vi "Diagram - Get All Text Refs.vi"(8 "error in (no error)":errorcluster, 11 "TopLevelDiagram in":refnum<vi>) -> (0 "error out":errorcluster, 2 "TextRefs":refnum<vi>[](array[refnum]), 3 "TopLevelDiagram out":refnum<vi>)   [LabVIEW 2017, in "csmHelper-Diagram.lvlib"]
doc: "-- <b>输入控件</b> --\n\n- <b>TopLevelDiagram in</b>:\n\n\n-- <b>输出控件</b> --\n\n- <b>TextRefs</b>:\n\n- <b>TopLevelDiagram out</b>:"
uses:
  csmHelper-Diagram.lvlib
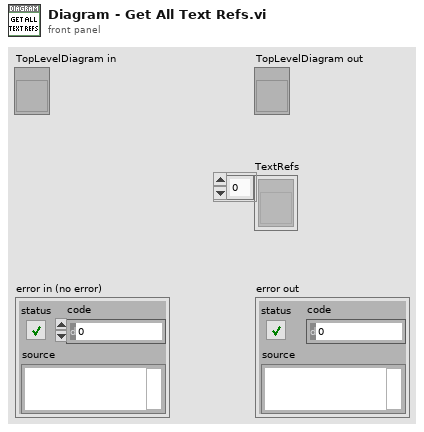
[diagram p1: front panel]
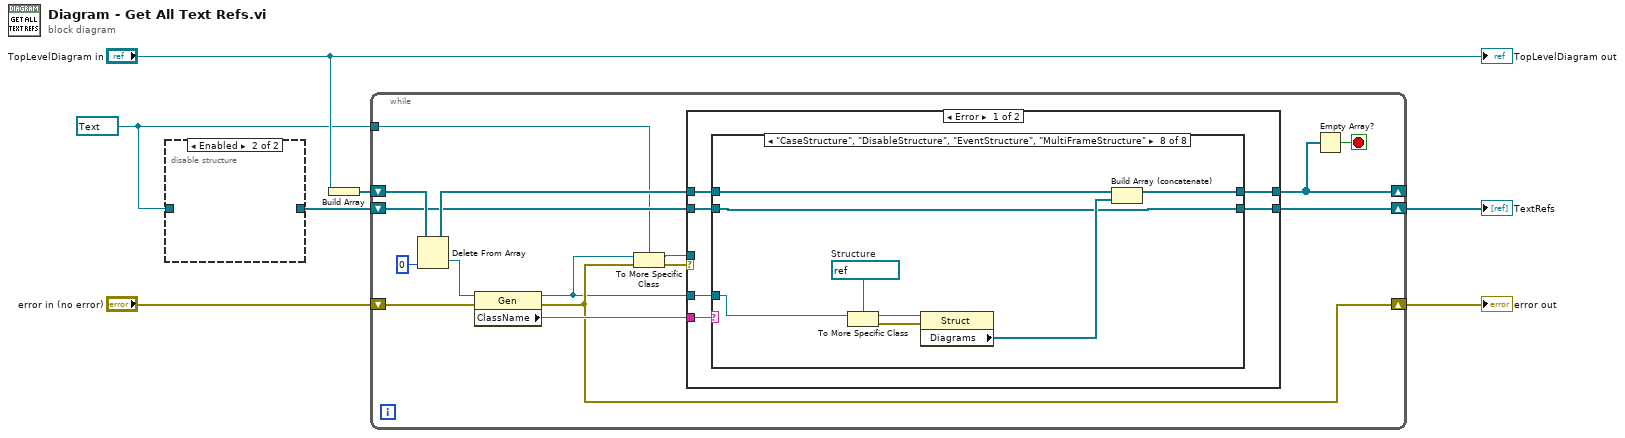
[diagram p0: block diagram]
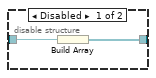
[diagram p2: hidden frame]
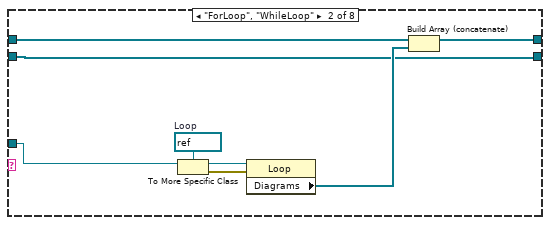
[diagram p4: hidden frame]
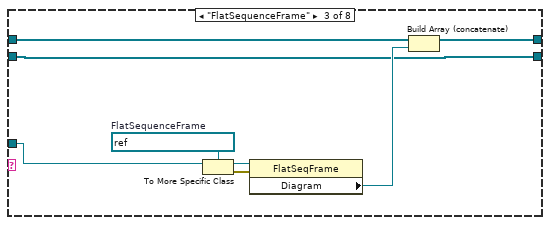
[diagram p5: hidden frame]
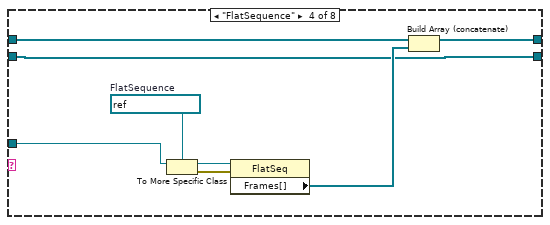
[diagram p6: hidden frame]
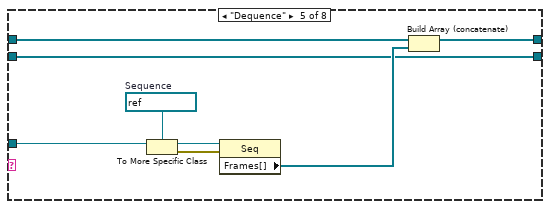
[diagram p7: hidden frame]
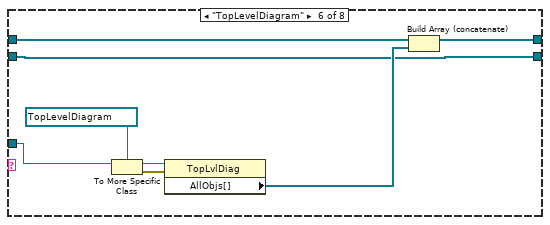
[diagram p8: hidden frame]
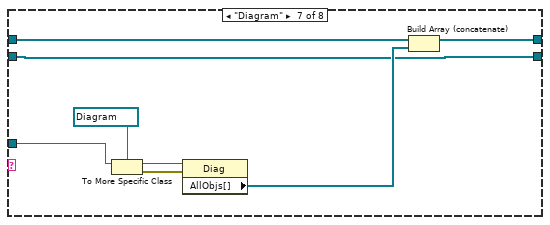
[diagram p9: hidden frame]
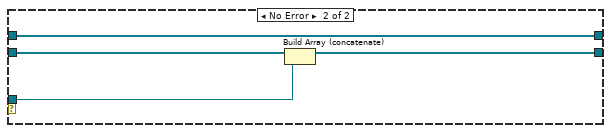
[diagram p10: hidden frame]
diagram:
  w1 = refnum<vi> refnum ("Refnum Type")
  n1 = disable-structure shown="Disabled" {
    disable-tunnel: [w8 _] -> w5
    disable-tunnel: w1 -> [w9 _]
    frame Disabled {
      n2 = Build Array(w9) -> (w8:refnum<vi>[])
    }
    frame Enabled {
    }
  }
  n3 = Build Array("TopLevelDiagram in") -> (w6:refnum<vi>[])
  n4 = while {
    shift-right: [w18] -> _
    shift-left: w6 -> [w23]
    shift-right: [w15] -> w4
    shift-left: w5 -> [w16]
    shift-right: [w14] -> w7
    shift-left: "error in (no error)" -> [w19]
    tunnel: w1 -> [w12]
    stop <- w24 stop-if-true
    n5 = Delete From Array(array=w23, index=0) -> (deleted portion=w21:refnum<vi>, array with subset deleted=w17:refnum<vi>[])  [unwired: 1 in]
    n6 = property class="Gen"(reference=w21, error in=w19) -> (reference out=w10:refnum<vi>, error out=w14:errorcluster, "ClassName"=w20:string)
    n7 = To More Specific Class(target class=w12, reference=w10, error in=w14) -> (specific class reference=w11:refnum<vi>, error out=w13:errorcluster)
    n8 = case shown="Error" w13 {
      tunnel: w20 -> [w30 _]
      tunnel: [w29 w92] -> w18
      tunnel: w17 -> [w28 w92]
      tunnel: w16 -> [w27 w91]
      tunnel: [w26 w90] -> w15
      tunnel: w11 -> [_ w89]
      tunnel: w10 -> [w25 _]
      frame Error {
        n9 = case shown="\"CaseStructure\", \"DisableStructure\", \"EventStructure\", \"MultiFrameStructure\"" w30 {
          tunnel: [w32 w36 w44 w53 w61 w69 w77 w85] -> w29
          tunnel: w28 -> [w32 w37 w45 w54 w62 w70 w78 w86]
          tunnel: w27 -> [w31 w34 w42 w51 w59 w67 w75 w83]
          tunnel: [w31 w34 w42 w51 w59 w67 w75 w83] -> w26
          tunnel: w25 -> [_ w33 w41 w49 w57 w65 w73 w81]
          frame "False", Default {
          }
          frame "ForLoop", "WhileLoop" {
            w38 = refnum<vi> refnum  # Loop
            n10 = To More Specific Class(target class=w38, reference=w33) -> (specific class reference=w39:refnum<vi>, error out=w40:errorcluster)  [unwired: 1 in]
            n11 = property class="Loop"(reference=w39, error in=w40) -> ("Diagrams"=w35:refnum<vi>[])  [unwired: 2 out]
            n12 = Build Array (concatenate)(w37, w35) -> (w36:refnum<vi>[])
          }
          frame "FlatSequenceFrame" {
            w46 = refnum<vi> refnum  # FlatSequenceFrame
            n13 = To More Specific Class(target class=w46, reference=w41) -> (specific class reference=w47:refnum<vi>, error out=w48:errorcluster)  [unwired: 1 in]
            n14 = property class="FlatSeqFrame"(reference=w47, error in=w48) -> ("Diagram"=w43:refnum<vi>)  [unwired: 2 out]
            n15 = Build Array (concatenate)(w45, w43) -> (w44:refnum<vi>[])
          }
          frame "FlatSequence" {
            w50 = refnum<vi> refnum  # FlatSequence
            n16 = To More Specific Class(target class=w50, reference=w49) -> (specific class reference=w55:refnum<vi>, error out=w56:errorcluster)  [unwired: 1 in]
            n17 = property class="FlatSeq"(reference=w55, error in=w56) -> ("Frames[]"=w52:refnum<vi>[])  [unwired: 2 out]
            n18 = Build Array (concatenate)(w54, w52) -> (w53:refnum<vi>[])
          }
          frame "Dequence" {
            w58 = refnum<vi> refnum  # Sequence
            n19 = To More Specific Class(target class=w58, reference=w57) -> (specific class reference=w63:refnum<vi>, error out=w64:errorcluster)  [unwired: 1 in]
            n20 = property class="Seq"(reference=w63, error in=w64) -> ("Frames[]"=w60:refnum<vi>[])  [unwired: 2 out]
            n21 = Build Array (concatenate)(w62, w60) -> (w61:refnum<vi>[])
          }
          frame "TopLevelDiagram" {
            n22 = To More Specific Class(target class=refnum<vi> refnum ("Block Diagram"), reference=w65) -> (specific class reference=w71:refnum<vi>, error out=w72:errorcluster)  [unwired: 1 in]
            n23 = property class="TopLvlDiag"(reference=w71, error in=w72) -> ("AllObjs[]"=w68:refnum<vi>[])  [unwired: 2 out]
            n24 = Build Array (concatenate)(w70, w68) -> (w69:refnum<vi>[])
          }
          frame "Diagram" {
            n25 = To More Specific Class(target class=refnum<vi> refnum ("Block Diagram"), reference=w73) -> (specific class reference=w79:refnum<vi>, error out=w80:errorcluster)  [unwired: 1 in]
            n26 = property class="Diag"(reference=w79, error in=w80) -> ("AllObjs[]"=w76:refnum<vi>[])  [unwired: 2 out]
            n27 = Build Array (concatenate)(w78, w76) -> (w77:refnum<vi>[])
          }
          frame "CaseStructure", "DisableStructure", "EventStructure", "MultiFrameStructure" {
            w82 = refnum<vi> refnum  # Structure
            n28 = To More Specific Class(target class=w82, reference=w81) -> (specific class reference=w87:refnum<vi>, error out=w88:errorcluster)  [unwired: 1 in]
            n29 = property class="Struct"(reference=w87, error in=w88) -> ("Diagrams"=w84:refnum<vi>[])  [unwired: 2 out]
            n30 = Build Array (concatenate)(w86, w84) -> (w85:refnum<vi>[])
          }
        }
      }
      frame No Error {
        n31 = Build Array (concatenate)(w91, w89) -> (w90:refnum<vi>[])
      }
    }
    n32 = Empty Array?(array=w18) -> (empty?=w24:bool)
  }
  "error out" <- w7
  "TextRefs" <- w4
  "TopLevelDiagram out" <- "TopLevelDiagram in"
